vi "Get Resource.vi"(8 "error in (no error)":errorcluster, 11 "Hardware Ref in":T1 format="%.0x") -> (0 "error out":errorcluster, 2 "Resource":string, 3 "Hardware Ref out":T1 format="%.0x", 4 "Found?":bool)   [LabVIEW 2017, in "Routing and Faulting Hardware API.lvlib"]
uses:
  Routing and Faulting Hardware API.lvlib
  <vilib>/NI Veristand/Custom Device API/Custom Device Item Ref.ctl
  <vilib>/NI Veristand/Custom Device API/Custom Device API.lvlib
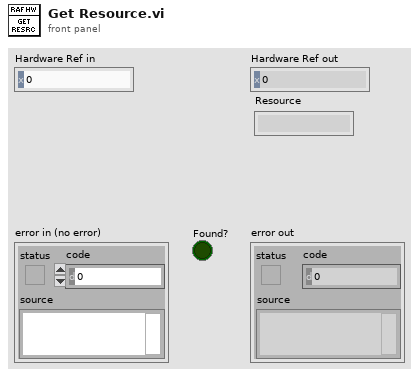
[diagram p1: front panel]
types:
  T1 = typedef "Custom Device API.lvlib/Custom Device Item Ref.ctl" = u64
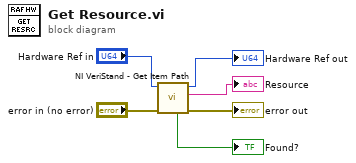
[diagram p0: block diagram]
diagram:
  n1 = call <vilib>:"NI VeriStand - Get Item Path.vi"("error in (no error)"="error in (no error)", "Item Ref in"="Hardware Ref in") -> ("error out"=→"error out":errorcluster, "Path"=→"Resource":string, "Item Ref out"=→"Hardware Ref out":T1, "Found"=→"Found?":bool)  [unwired: 6 in]
